vi "New Batch.vi"(8 "error out 2":errorcluster, 9 "Batch Data 3":T1, 10 "Batch data":string[](array[string]), 11 "Module Number  3":dbl=1.0) -> (0 "error out":errorcluster, 3 "Sucess ?":bool)   [LabVIEW 2015, in "Copy of Untitled Library 1.lvlib"]
uses:
  Copy of Untitled Library 1.lvlib
  Controls/Caller Queue Control .ctl
  Controls/Control 1.ctl
  Controls/Enum Constant.ctl
  <userlib>/origin_lib_main/db_interface/DB Operations Enum.ctl
  <userlib>/origin_lib_main/db_interface/DB Interface.lvlib
panel:
  in  "Cluster":T2
  out "concatenated string":string
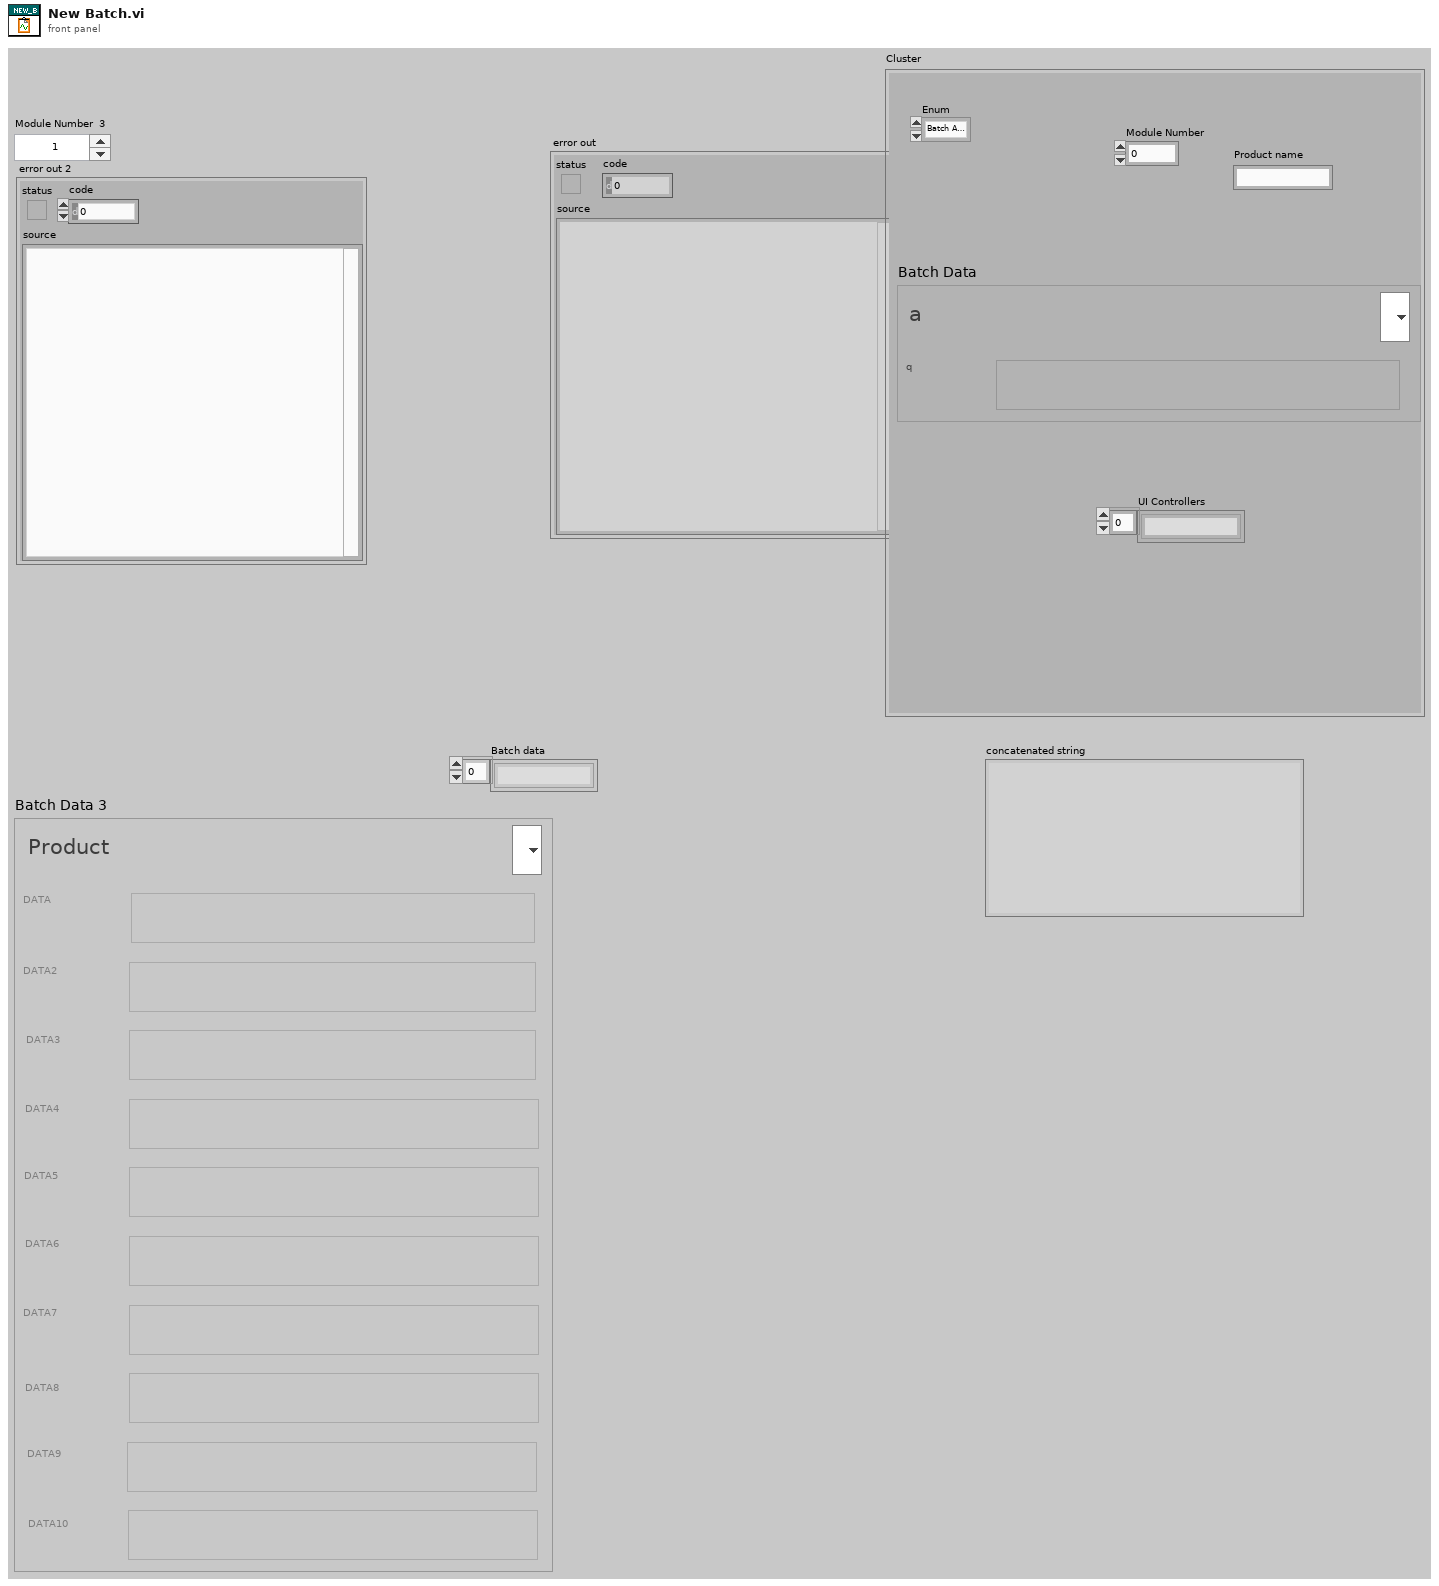
[diagram p1: front panel]
types:
  T1 = typedef "Copy of Untitled Library 1.lvlib/Control 1.ctl" = cluster{"DATA":string, "DATA 2":string, "DATA 3":string, "DATA 4":string, "DATA 5":string, "DATA 6":string, "DATA 7":string, "DATA 8":string, "DATA 9":string, "DATA 10":string, "Product":string}
  T2 = typedef "Caller Queue Control .ctl" = cluster{"Enum":enum16{"Batch Added", "Batch Deleted", "Batch Opened", "Batch Closed", "Batch Edited", "new Product Added", "Product deleted "}, "Batch Data 3":T1, "UI Controllers":string[], "Product name":string, "Module Number":dbl}
  T3 = typedef "DB Interface.lvlib/DB Operations Enum.ctl" = enum16{"Select", "Update", "Insert", "Delete", "Fetch SQL Query", "Execute SQL Query", "Drop Table", "List Tables"}
  T4 = typedef "Enum Constant.ctl" = enum16{"Init", "Read", "Write"}
  T5 = typedef "FGV Data.ctl" = T6[]
  T6 = typedef "FGV Cluster Data.ctl" = cluster{"Manual/Automatic":bool, "UI Controllers ":string[], "UI Primery Key ":dbl[], "Caller Queue & MSG":T7, "Module ID":dbl, "DB Reference In":T8, "Products Columns":string[], "Cluster":cluster{"Delete Product":enum8{"Enabled", "Disabled", "Disabled and Grayed Out"}, "Add Product ":enum8{"Enabled", "Disabled", "Disabled and Grayed Out"}, "EDIT BATCH":enum8{"Enabled", "Disabled", "Disabled and Grayed Out"}, "Open Batch ":enum8{"Enabled", "Disabled", "Disabled and Grayed Out"}, "Close Batch":enum8{"Enabled", "Disabled", "Disabled and Grayed Out"}, "Delete Batch":enum8{"Enabled", "Disabled", "Disabled and Grayed Out"}, "Add Batch ":enum8{"Enabled", "Disabled", "Disabled and Grayed Out"}}}
  T7 = typedef "Queue and Caller MSG.ctl" = cluster{"Caller Queue":refnum<queue>, "Caller MSG":string}
  T8 = typedef "NI_Database_API.lvlib/Conn ObjectReference.ctl" = refnum<k1>
  T9 = enum16{"Batch Added", "Batch Deleted", "Batch Opened", "Batch Closed", "Batch Edited", "new Product Added", "Product deleted "}
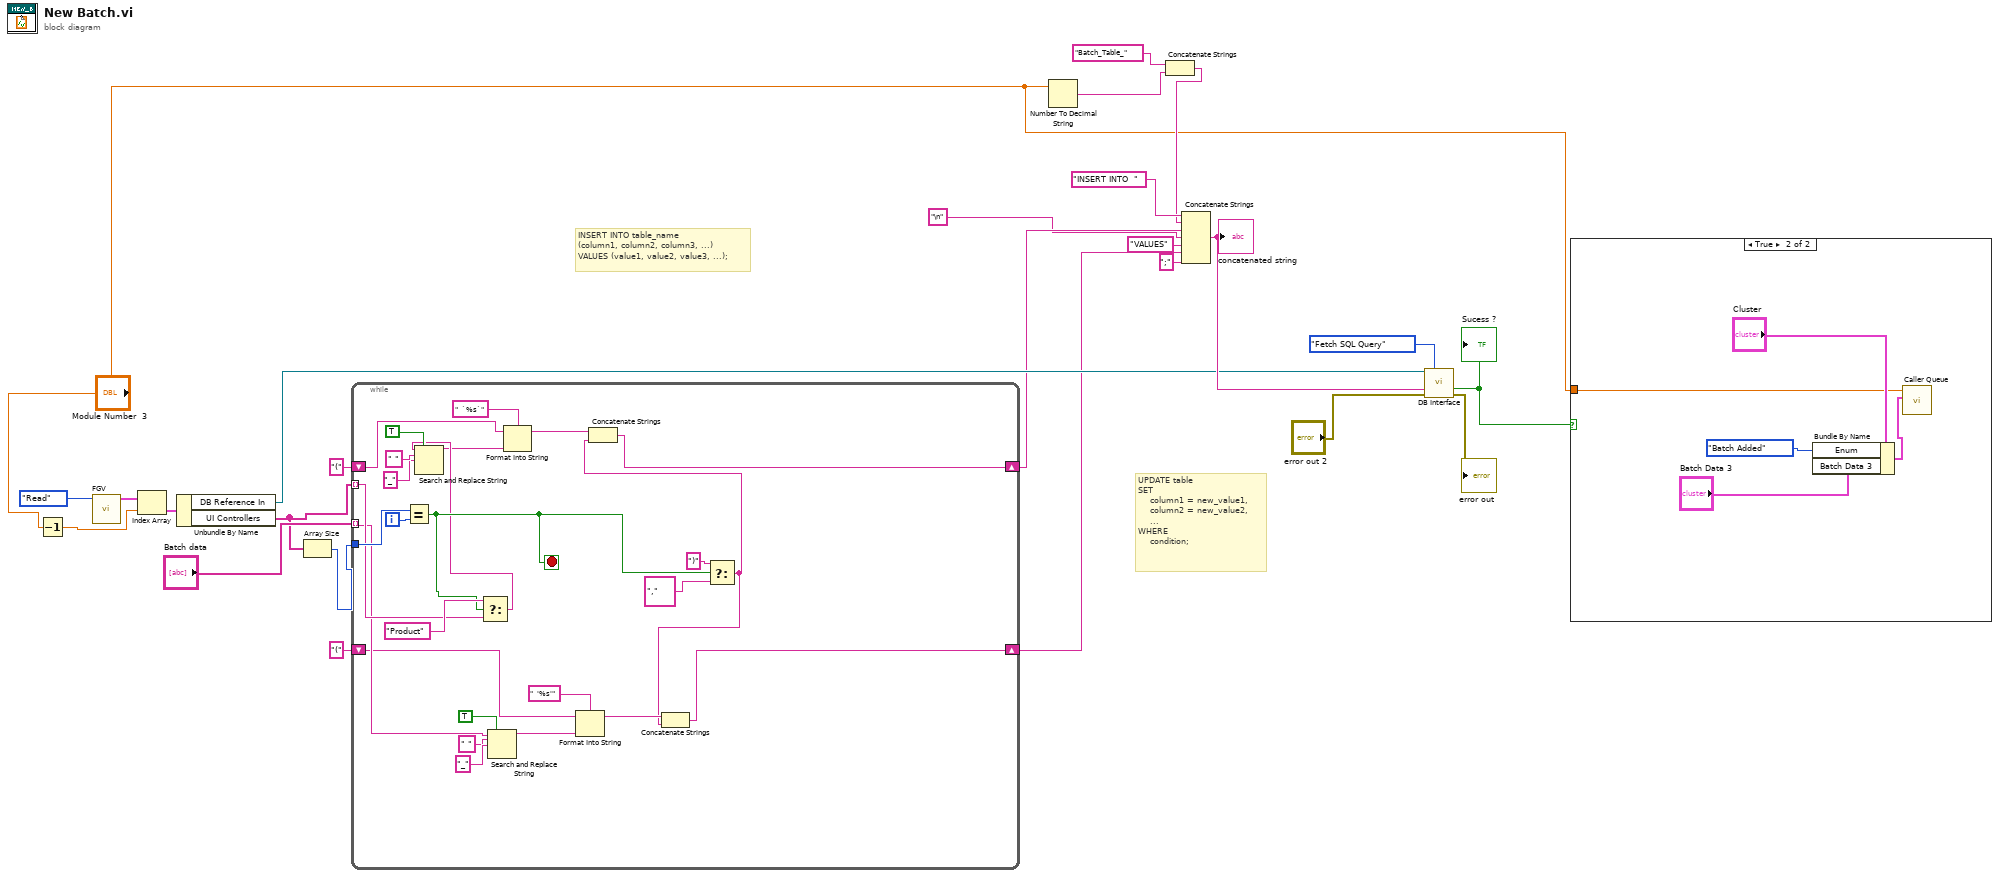
[diagram p0: block diagram]
diagram:
  # "UPDATE table\nSET \n    column1 = new_value1,\n    column2 = new_value2,\n    ...\nWHERE\n    condition;"
  # "INSERT INTO table_name \n(column1, column2, column3, ...)\nVALUES (value1, value2, value3, ...);"
  n1 = Decrement(x="Module Number  3") -> (x-1=w21:dbl)
  n2 = call "FGV.vi"("Enum"=Enum_Constant."Read") -> ("Read Data"=w23:T5)  [unwired: 9 in, 1 out]
  n3 = Index Array(array=w23, index=w21) -> (element=w24:T6)
  n4 = Unbundle By Name(w24) -> ("DB Reference In"=w14:T8, "UI Controllers"=w12:string[])
  n5 = Array Size(array=w12) -> (size(s)=w10:i32)
  n6 = while {
    shift-right: [w42] -> w9
    shift-left: "(" -> [w30]
    tunnel: w10 -> [w46]
    tunnel: w12 -> [w39] mode=indexing
    tunnel: "Batch data" -> [w29] mode=indexing
    shift-right: [w27] -> w7
    shift-left: "(" -> [w26]
    i -> [w47]
    stop <- w40 stop-if-true
    n7 = Equal?(x=w46, y=w47) -> (x = y?=w40:bool)
    n8 = Select(t="Product", s=w40, f=w39) -> (s? t:f=w38:string)
    n9 = Search and Replace String(replace all?=TRUE ("replace all? (F)"), input string=w38, search string=" ", replace string="_" ("replace string (\"\")")) -> (result string=w37:string)  [unwired: 4 in, 3 out]
    n10 = Search and Replace String(replace all?=TRUE ("replace all? (F)"), input string=w29, search string=" ", replace string="_" ("replace string (\"\")")) -> (result string=w36:string)  [unwired: 4 in, 3 out]
    n11 = Format Into String(format string="  `%s`", initial string=w30, w37) -> (resulting string=w50:string)  [unwired: 1 in, 1 out]
    n12 = Format Into String(format string="  '%s'", initial string=w26, w36) -> (resulting string=w32:string)  [unwired: 1 in, 1 out]
    n13 = Select(t=")", s=w40, f=",") -> (s? t:f=w28:string)
    n14 = Concatenate Strings(w50, w28) -> (w42:string)
    n15 = Concatenate Strings(w32, w28) -> (w27:string)
  }
  n16 = Number To Decimal String(number="Module Number  3") -> (decimal integer string=w19:string)  [unwired: 1 in]
  n17 = Concatenate Strings("Batch_Table_" ("string"), w19) -> (w18:string)
  n18 = Concatenate Strings("INSERT INTO  " ("string"), w18, w9, "\n" ("string"), "VALUES" ("string"), w7, ";" ("string")) -> (w16:string)
  "concatenated string" <- w16
  n19 = call <userlib>:"DB Interface.vi"("DB Ref In"=w14, "Operation"=DB_Operations_Enum."Fetch SQL Query", "SQL Query"=w16, "error in (no error)"="error out 2") -> ("Sucess ?"=w1:bool, "error out"=→"error out":errorcluster)  [unwired: 8 in, 2 out]
  "Sucess ?" <- w1
  n20 = case shown="True" w1 {
    tunnel: "Module Number  3" -> [_ w54]
    frame False {
    }
    frame True {
      n21 = Bundle By Name(cluster="Cluster", "Enum"=T9."Batch Added", "Batch Data 3"="Batch Data 3") -> (w52:T2)
      n22 = call "Caller Queue .vi"("Cluster"=w52, "Module Number  3"=w54) -> ()  [unwired: 9 in, 1 out]
    }
  }
